vi "PlaceDataInControls.vi"(7 "TipStrip":string, 8 "error in (no error)":errorcluster, 9 "Variant":variant, 10 "DataArray":string[](array[string]), 11 "ControlNamesArray":string[](array[string])) -> (0 "error out":errorcluster)   [LabVIEW 2016, in "M1M3SupportEUI_Views.lvlib"]
uses:
  M1M3SupportEUI_Views.lvlib
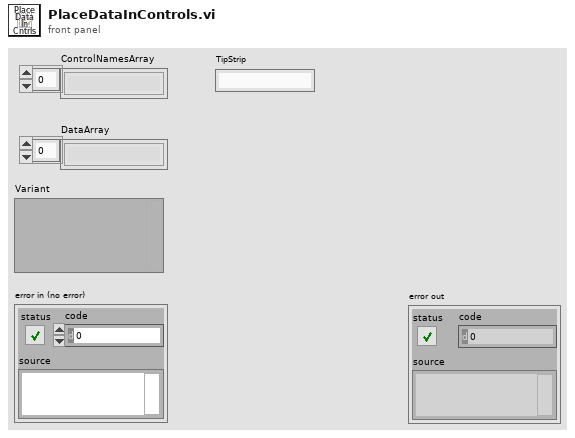
[diagram p1: front panel]
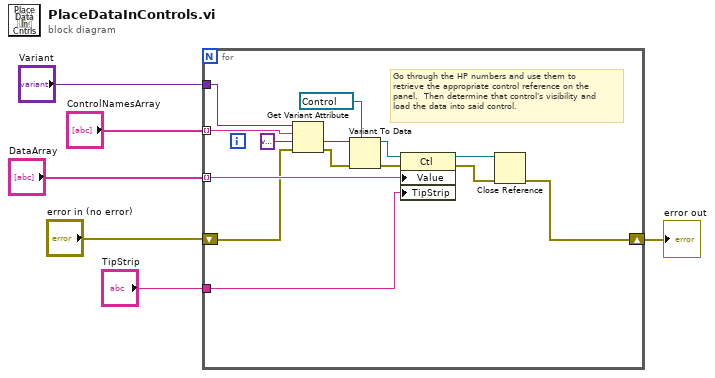
[diagram p0: block diagram]
diagram:
  n1 = for {
    tunnel: "DataArray" -> [w16] mode=indexing
    shift-right: [w9] -> w2
    shift-left: "error in (no error)" -> [w12]
    tunnel: "Variant" -> [w20]
    tunnel: "ControlNamesArray" -> [w11] mode=indexing
    tunnel: "TipStrip" -> [w7]
    # "Go through the HP numbers and use them to \nretrieve the appropriate control reference on the\npanel.  Then determine that control's visibility and\nload the data into said control."
    n2 = Get Variant Attribute(Variant=w20, name=w11, default value (empty Variant)=variant ("default value (empty variant)"), error in=w12) -> (value=w17:variant, error out=w15:errorcluster)  [unwired: 2 out]
    n3 = Variant To Data(error in=w15, type=refnum<vi> refnum ("reference out"), Variant=w17) -> (data=w14:refnum<vi>, error out=w13:errorcluster)
    n4 = property class="Ctl"(reference=w14, error in=w13, "Value"=w16, "TipStrip"=w7) -> (reference out=w8:refnum<vi>, error out=w10:errorcluster)
    n5 = Close Reference(reference=w8, error in (no error)=w10) -> (error out=w9:errorcluster)
  }
  "error out" <- w2
